vi "Create.vi"(8 "error in (no error)":errorcluster, 11 "obj":refnum<class "SciWare_ByRefActiveObj_V1.0.0.lvclass">) -> (0 "error out":errorcluster, 3 "obj out":refnum<class "SciWare_ByRefActiveObj_V1.0.0.lvclass">)   [LabVIEW 2009, in "SciWare_ByRefActiveObj_V1.0.0.lvclass"]
doc: "Creates an active by ref object.\n\nBSD License (http://www.opensource.org/licenses/bsd-license.php)"
uses:
  SciWare_ByRefActiveObj_V1.0.0.lvclass
  Private/DataMembers.ctl
  SciWare_ByRefActiveObj_V1.0.0.lvclass/SciWare_ByRefActiveObj_V1.0.0.ctl
panel:
  in  "data members (type)":T1
  # "BSD License (http://www.opensource.org/licenses/bsd-license.php)"
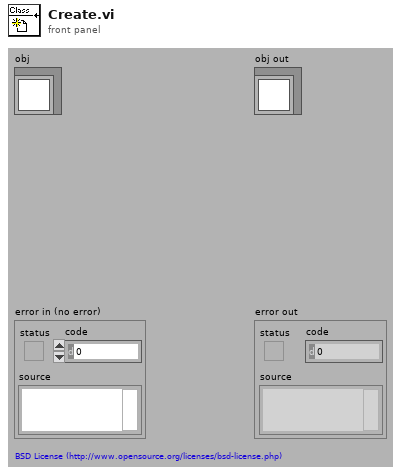
[diagram p1: front panel]
types:
  T1 = typedef "SciWare_ByRefActiveObj_V1.0.0.lvclass/DataMembers.ctl" = cluster{"String":string}
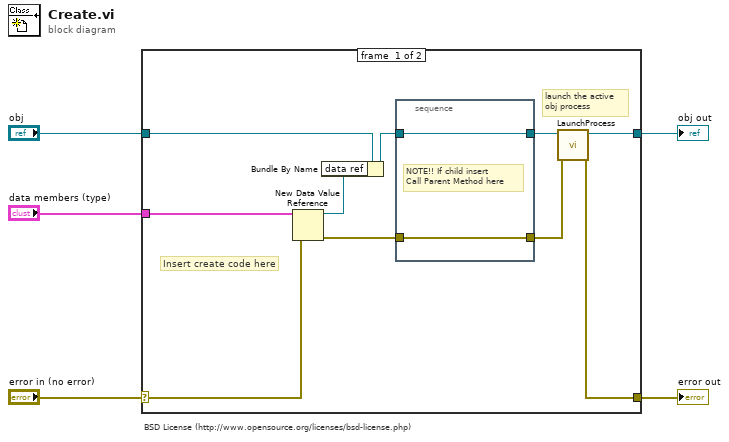
[diagram p0: block diagram]
diagram:
  # "BSD License (http://www.opensource.org/licenses/bsd-license.php)"
  n1 = case shown="No Error" "error in (no error)" {
    selector: "error in (no error)" -> [w15 w19]
    tunnel: [w13 w19] -> w4
    tunnel: "data members (type)" -> [w12 _]
    tunnel: [w11 w18] -> w2
    tunnel: "obj" -> [w10 w18]
    frame #0 {
      # "Insert create code here"
      # "launch the active\nobj process"
      n2 = New Data Value Reference(data value=w12, error in=w15) -> (data value reference=w14:refnum<data-value>, error out=w7:errorcluster)
      n3 = Bundle By Name(cluster=w10, "data ref"=w14) -> (w9:refnum<class "SciWare_ByRefActiveObj_V1.0.0.lvclass">)
      n4 = stacked-sequence {
        tunnel: [w17] -> w8
        tunnel: w9 -> [w17]
        tunnel: w7 -> [w16]
        tunnel: [w16] -> w6
        frame #0 {
          # "NOTE!! If child insert\nCall Parent Method here"
        }
      }
      n5 = call-dynamic "LaunchProcess.vi"("error in (no error)"=w6, "obj"=w8) -> ("error out"=w13:errorcluster, "obj out"=w11:refnum<class "SciWare_ByRefActiveObj_V1.0.0.lvclass">)  [unwired: 8 in]
    }
    frame #1 {
    }
  }
  "error out" <- w4
  "obj out" <- w2
